vi "TDC_getLastTimestamps.vi"(8 "Error In":errorcluster, 10 "Buffer Size":i32, 11 "Reset":bool) -> (0 "Error Out":errorcluster, 1 "Channel Numbers":i8[](array[numeric]), 2 "Timestamps":i64[](array[numeric]), 3 "Valid Data":i32)   [LabVIEW 2011]
uses:
  tdcbase.dll
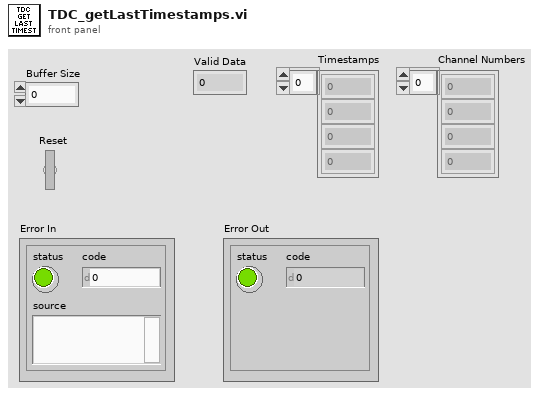
[diagram p1: front panel]
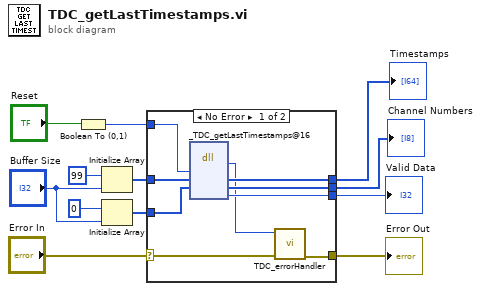
[diagram p0: block diagram]
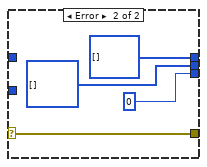
[diagram p2: hidden frame]
diagram:
  n1 = Boolean To (0,1)(Boolean="Reset") -> (0, 1=w6:i16)
  n2 = Initialize Array(i64 99, "Buffer Size") -> (w8:i64[])
  n3 = Initialize Array(i8 0, "Buffer Size") -> (w2:i8[])
  n4 = case shown="No Error" "Error In" {
    selector: "Error In" -> [w15 w25]
    tunnel: [w14 w25] -> w11
    tunnel: [w21 i64[] []] -> w10
    tunnel: w8 -> [w20 _]
    tunnel: w6 -> [w19 _]
    tunnel: [w18 0] -> w5
    tunnel: w2 -> [w17 _]
    tunnel: [w16 i8[] []] -> w1
    frame No Error {
      n5 = dll-call lib="X:/tdcbase.dll" fn="_TDC_getLastTimestamps@16"("reset"=w19, "timestamps"=w20, "channels"=w17) -> ("return type"=w13:i32, "timestamps"=w21:i64[], "channels"=w16:i8[], "valid"=w18:i32)  [unwired: 5 in, 2 out]
      n6 = call "TDC_errorHandler.vi"("Error In"=w15, "TDC Return Code"=w13) -> ("Error Out"=w14:errorcluster)  [unwired: 9 in]
    }
    frame Error {
    }
  }
  "Error Out" <- w11
  "Timestamps" <- w10
  "Valid Data" <- w5
  "Channel Numbers" <- w1
